vi "get enums.vi"() -> ()   [LabVIEW 2013]
uses:
  C:/Program Files/Princeton Instruments/LightField/PrincetonInstruments.LightFieldAddInSupportServices.dll
  Program Files/Princeton Instruments/LightField/PrincetonInstruments.LightFieldAddInSupportServices.dll
panel:
  out "data":i32[](array[numeric])
  out "GetNames":string[](array[string])
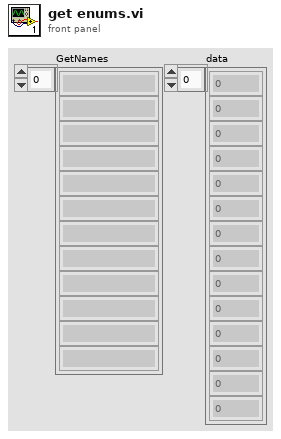
[diagram p1: front panel]
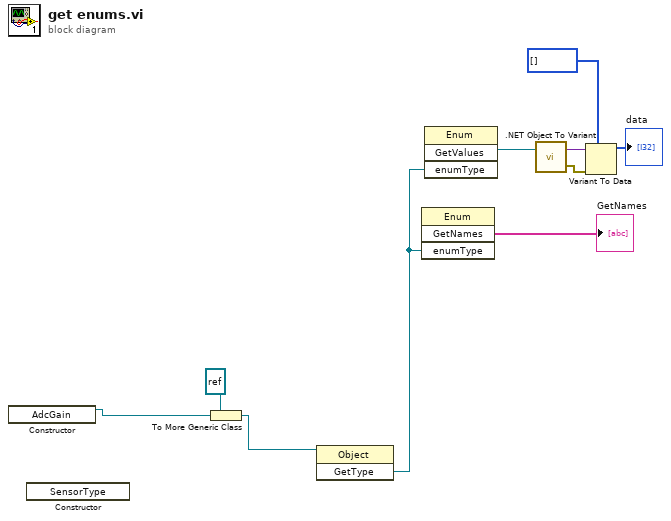
[diagram p0: block diagram]
diagram:
  n1 = constructor class="AdcGain"() -> (reference out=w1:refnum<k24>)  [unwired: 3 in, 2 out]
  n2 = constructor class="SensorType"() -> ()  [unwired: 3 in, 3 out]
  n3 = To More Generic Class(target class=refnum<k24> refnum, reference=w1) -> (generic class reference=w3:refnum<k24>)
  n4 = invoke class="Object" method="GetType"(reference=w3) -> ("GetType"=w9:refnum<k24>)  [unwired: 2 in, 2 out]
  n5 = invoke class="Enum" method="GetNames"("enumType"=w9) -> ("GetNames"=→"GetNames":string[])  [unwired: 3 in, 3 out]
  n6 = invoke class="Enum" method="GetValues"("enumType"=w9) -> ("GetValues"=w8:refnum<k24>)  [unwired: 3 in, 3 out]
  n7 = call <vilib>:".NET Object To Variant.vi"(".NET object"=w8) -> ("error out"=w7:errorcluster, "variant"=w6:variant)  [unwired: 1 in]
  n8 = Variant To Data(error in=w7, type=i32[] [], Variant=w6) -> (data=→"data":i32[])  [unwired: 1 out]
